vi "read_NI.vi"(6 "error in":errorcluster, 11 "fpga-ref-in":refnum<k20>) -> (0 "all_pds":dbl[](array[numeric]), 1 "-pd3/pd1":dbl, 2 "pd3/pd1":dbl, 3 "fpga-ref-out":refnum<k20>, 4 "error out":errorcluster)   [LabVIEW 2024]
uses:
  <vilib>/FPGAPlugInAG/NI 9147/niLvFpga_Open_NI 9147.vi
  <vilib>/rvi/interface/common/dynamic/niFpgaDynamicAddResources.vi
  <vilib>/FPGAPlugInAG/Dynamic/niLvFpga_Run_Dynamic.vi
  <vilib>/Utility/error.llb/Error Cluster From Error Code.vi
  <vilib>/rvi/errors/niLvFpgaAdjustHostInterfaceError.vi
  <vilib>/FPGAPlugInAG/Dynamic/niLvFpga_Close_Dynamic.vi
  <vilib>/rvi/interface/nirviOpenFPGA/nirviOpenFPGA.xnode
  FPGA Bitfiles/dircdaq-automate_FPGATarget_fpga_RyAY8MzD2n8.lvbitx
  fpga.vi
  <vilib>/rvi/interface/nirviMethod/nirviMethod.xnode
  <vilib>/rvi/interface/nirviReadWriteControl/nirviReadWriteControl.xnode
  <vilib>/rvi/interface/nirviCloseFPGA/nirviCloseFPGA.xnode
  NiFpgaLv.dll
  <vilib>/rvi/interface/Simulation/niFpgaSimulationCallBeginRW.vi
  <vilib>/Analysis/NI_AALBase.lvlib
panel:
  out "pd2/pd1":dbl
  out "ch2-sd":dbl format="%^#_6g"
  out "ch2-avg":dbl format="%^#_6g"
  out "ch1-sd":dbl format="%^#_6g"
  out "ch1-avg":dbl format="%^#_6g"
  out "ch0-sd":dbl format="%^#_6g"
  out "ch0-avg":dbl format="%^#_6g"
  out "fpga-heartbeat":bool
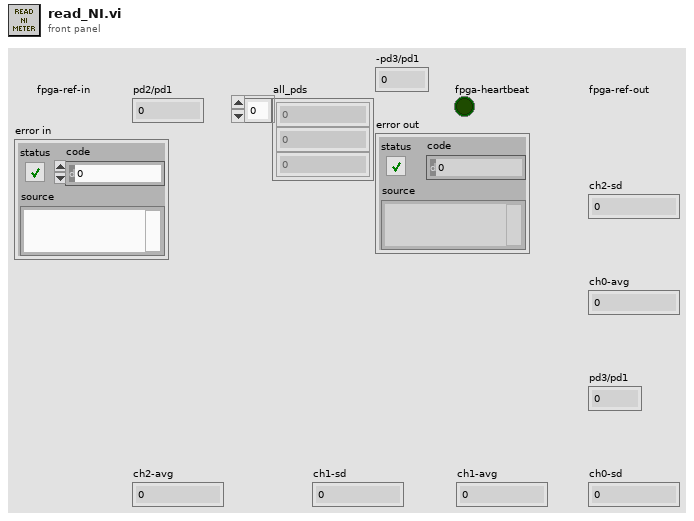
[diagram p1: front panel]
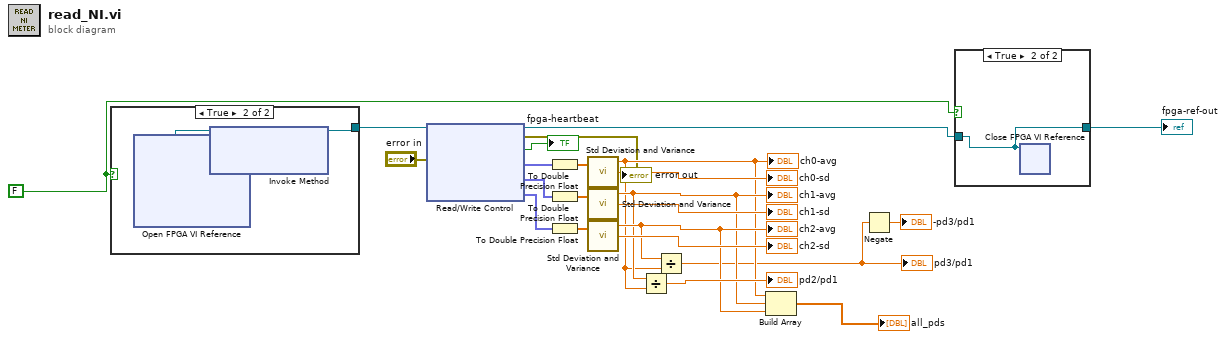
[diagram p0: block diagram]
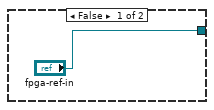
[diagram p3: hidden frame]
diagram:
  w3 = FALSE ("dev mode = T")
  n1 = case shown="True" w3 {
    tunnel: ["fpga-ref-in" w25] -> w4
    frame False {
    }
    frame True {
      n2 = xnode "Open FPGA VI Reference"() -> ("FPGA VI Reference Out"=w26:refnum<k20>)  [unwired: 2 in, 1 out]
      n3 = xnode "Invoke Method"("FPGA VI Reference In"=w26) -> ("FPGA VI Reference Out"=w25:refnum<k20>)  [unwired: 2 in, 1 out]
    }
  }
  n4 = xnode "Read/Write Control"("FPGA VI Reference In"=w4, "error in"="error in") -> ("FPGA VI Reference Out"=w2:refnum<k20>, "error out"=→"error out":errorcluster, "fpga-heartbeat"=→"fpga-heartbeat":bool, "ch0"=w9:fxp<+/-,32,-1>[], "ch1"=w12:fxp<+/-,32,-1>[], "ch2"=w14:fxp<+/-,32,-1>[])
  n5 = To Double Precision Float(number=w9) -> (double precision float=w11:dbl[])
  n6 = To Double Precision Float(number=w12) -> (double precision float=w10:dbl[])
  n7 = To Double Precision Float(number=w14) -> (double precision float=w13:dbl[])
  n8 = call <vilib>:"Std Deviation and Variance.vi"("X"=w11) -> ("mean"=w16:dbl, "standard deviation"=→"ch0-sd":dbl)  [unwired: 1 in, 1 out]
  "ch0-avg" <- w16
  n9 = call <vilib>:"Std Deviation and Variance.vi"("X"=w10) -> ("mean"=w18:dbl, "standard deviation"=→"ch1-sd":dbl)  [unwired: 1 in, 1 out]
  "ch1-avg" <- w18
  n10 = call <vilib>:"Std Deviation and Variance.vi"("X"=w13) -> ("mean"=w19:dbl, "standard deviation"=→"ch2-sd":dbl)  [unwired: 1 in, 1 out]
  "ch2-avg" <- w19
  n11 = Divide(x=w18, y=w16) -> (x/y=→"pd2/pd1":dbl)
  n12 = Divide(x=w19, y=w16) -> (x/y=w7:dbl)
  "pd3/pd1" <- w7
  n13 = Build Array(w16, w18, w19) -> (→"all_pds":dbl[])
  n14 = Negate(x=w7) -> (-x=→"-pd3/pd1":dbl)
  n15 = case shown="True" w3 {
    tunnel: w2 -> [w27 w28]
    tunnel: [w27 w28] -> w1
    frame False {
    }
    frame True {
      n16 = xnode "Close FPGA VI Reference"("FPGA VI Reference In"=w28) -> ()  [unwired: 1 in, 1 out]
    }
  }
  "fpga-ref-out" <- w1
